vi "dfd_DFXPSimu AccAdd (scaler).vi"(5 "quantize output? (T)":bool=TRUE, 7 "op params":T2={"source"=0, "is floating?"=FALSE, "o-mode"=enum."Wrap", "q-mode"=enum."Truncation", "wl"=1, "high limit"=0, "low limit"=0, "iwl"=0, "sign?"=TRUE} {"source" items=["Coef a/k"=0, "Coef b/v"=7, "Input"=1, "Output"=2, "Multiplicand"=3, "Product"=4, "Sum"=5, "Delay"=6, "Gain"=8]}, 8 "filtering statistics in":T6(array[cluster]) {"statistics information"."min value" format="%.2f"; "statistics information"."max value" format="%.2f"; "Quantizer Source" items=["Coefficients a/k"=0, "Coefficients b/v"=7, "Input"=1, "Output"=2, "Multiplicand"=3, "Product"=4, "Sum"=5, "Delay"=6]}, 10 "addend":T1={"value"=0, "wl"=0, "iwl"=0, "Signed"=TRUE} {"value" format="%.0x"}, 11 "acc in":T1={"value"=0, "wl"=0, "iwl"=0, "Signed"=TRUE} {"value" format="%.0x"}) -> (0 "filtering statistics out":T6(array[cluster]) {"statistics information"."min value" format="%.2f"; "statistics information"."max value" format="%.2f"; "Quantizer Source" items=["Coefficients a/k"=0, "Coefficients b/v"=7, "Input"=1, "Output"=2, "Multiplicand"=3, "Product"=4, "Sum"=5, "Delay"=6]}, 3 "acc out":T1={"value"=0, "wl"=0, "iwl"=0, "Signed"=TRUE} {"value" format="%.0x"})   [LabVIEW 2017, in "NI_DigFilter_FXP.lvlib"]
uses:
  <vilib>/addons/Digital Filter Design/NI_DigFilter_FXP.lvlib
  <vilib>/addons/Digital Filter Design/_Objects.llb/dfd_DFXP Data Type (scaler).ctl
  <vilib>/addons/Digital Filter Design/_Objects.llb/DFD Quantization Sources.ctl
  <vilib>/addons/Digital Filter Design/_Objects.llb/DFD FXP Statistics Data.ctl
  <vilib>/addons/Digital Filter Design/_Objects.llb/dfd_DFXP Operation Parameter.ctl
  <vilib>/addons/Digital Filter Design/_Objects.llb/dfd_Internal Quantization Srcs.ctl
  <vilib>/addons/Digital Filter Design/NI_DigFilterLicensed.lvlib
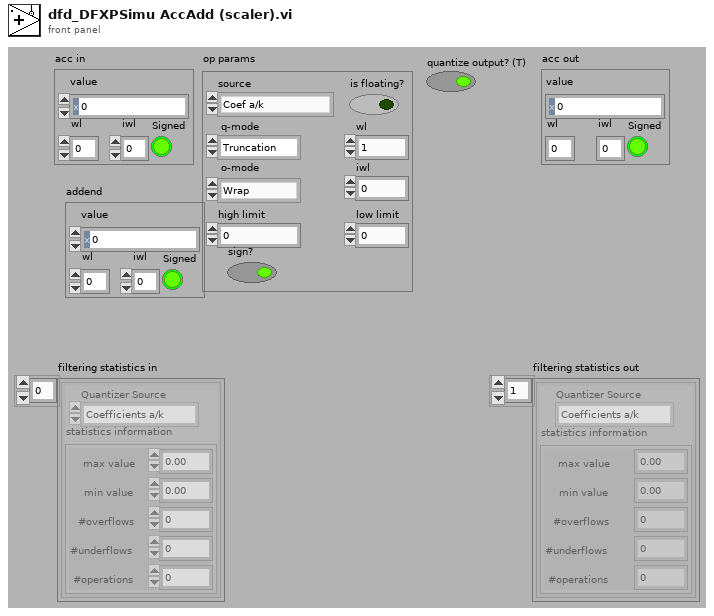
[diagram p1: front panel]
types:
  T1 = typedef "dfd_DFXP Data Type (scaler).ctl" = cluster{"value":i64, "wl":i16, "iwl":i16, "Signed":bool}
  T2 = typedef "dfd_DFXP Operation Parameter.ctl" = cluster{"source":T3, "is floating?":bool, "o-mode":enum16{"Saturation", "Wrap"}, "q-mode":enum16{"Nearest", "Truncation"}, "wl":i16, "high limit":i64, "low limit":i64, "iwl":i16, "sign?":bool}
  T3 = typedef "NI_DigFilterLicensed.lvlib/dfd_Internal Quantization Srcs.ctl" = u16
  T4 = typedef "NI_DigFilterLicensed.lvlib/DFD Quantization Sources.ctl" = u16
  T5 = typedef "NI_DigFilterLicensed.lvlib/DFD FXP Statistics Data.ctl" = cluster{"max value":ext, "min value":ext, "#overflows":i32, "#underflows":i32, "#operations":i32}
  T6 = cluster{"Quantizer Source":T4, "statistics information":T5}[]
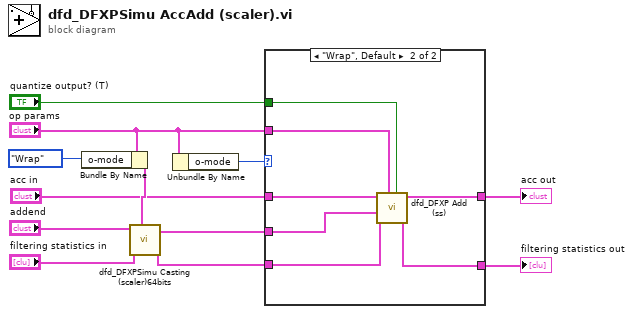
[diagram p0: block diagram]
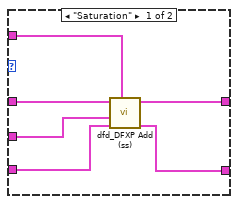
[diagram p2: hidden frame]
diagram:
  n1 = Bundle By Name(cluster="op params", "o-mode"=enum16{"Saturation", "Wrap"}."Wrap" ("o_mode")) -> (w11:T2)
  n2 = call <vilib>:"dfd_DFXPSimu Casting (scaler)64bits.vi"("op params"=w11, "filtering statistics in"="filtering statistics in", "Value in"="addend") -> ("filtering statistics out"=w6:T6, "Value out"=w3:T1)  [unwired: 1 in, 6 out]
  n3 = Unbundle By Name("op params") -> ("o-mode"=w9:enum16{"Saturation", "Wrap"})
  n4 = case shown="\"Wrap\", Default" w9 {
    tunnel: "quantize output? (T)" -> [_ w25]
    tunnel: "op params" -> [w18 w24]
    tunnel: w3 -> [w14 w19]
    tunnel: w6 -> [w17 w23]
    tunnel: [w16 w21] -> w5
    tunnel: [w15 w22] -> w4
    tunnel: "acc in" -> [w13 w20]
    frame "Saturation" {
      n5 = call <vilib>:"dfd_DFXP Add (ss).vi"("op params"=w18, "filtering statistics in"=w17, "Value in 2"=w14, "Value in"=w13) -> ("filtering statistics out"=w15:T6, "Value out"=w16:T1)  [unwired: 1 in, 5 out]
    }
    frame "Wrap", Default {
      n6 = call <vilib>:"dfd_DFXP Add (ss).vi"("quantize output? (T)"=w25, "op params"=w24, "filtering statistics in"=w23, "Value in 2"=w19, "Value in"=w20) -> ("filtering statistics out"=w22:T6, "Value out"=w21:T1)  [unwired: 5 out]
    }
  }
  "filtering statistics out" <- w4
  "acc out" <- w5
